vi "FlatToRichnixnet_grpc_DbMergeRequest.vi"(5 "OutputClusterType":T1, 11 "InputCluster":T3) -> (3 "OutputCluster":T1)   [LabVIEW 2025, in "xnet-grpc_client.lvlib"]
uses:
  nixnet_grpc_DbMergeRequest_Flat.ctl
  nidevice_grpc_Session_Flat.ctl
  nixnet_grpc_CopyMode.ctl
  nixnet_grpc_DbMergeRequest.ctl
  nixnet_grpc_DbMergeRequest_copy_mode_enum/nixnet_grpc_DbMergeRequest_copy_mode_enum.lvclass
  nidevice_grpc_Session.ctl
  xnet-grpc_client.lvlib
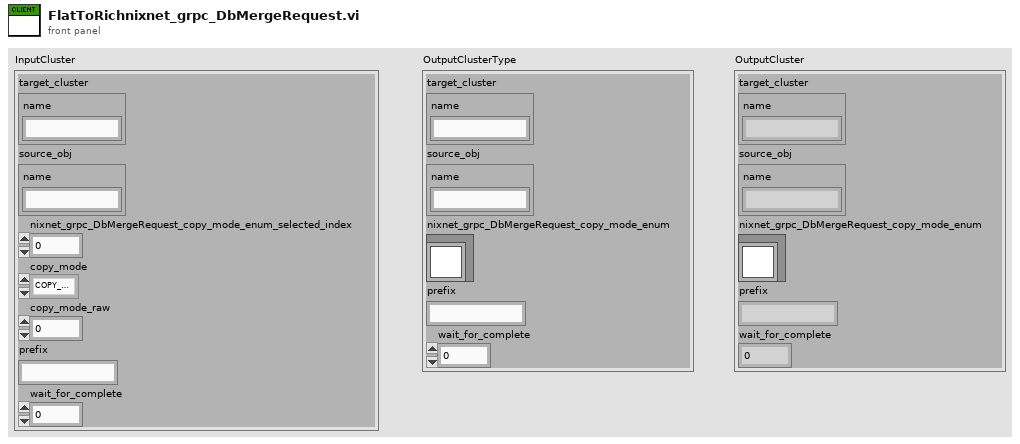
[diagram p1: front panel]
types:
  T1 = typedef "xnet-grpc_client.lvlib/nixnet_grpc_DbMergeRequest.ctl" = cluster{"target_cluster":T2, "source_obj":T2, "nixnet_grpc_DbMergeRequest_copy_mode_enum":refnum<class "nixnet_grpc_DbMergeRequest_copy_mode_enum.lvclass">, "prefix":string, "wait_for_complete":u32}
  T2 = typedef "xnet-grpc_client.lvlib/nidevice_grpc_Session.ctl" = cluster{"name":string}
  T3 = typedef "xnet-grpc_client.lvlib/nixnet_grpc_DbMergeRequest_Flat.ctl" = cluster{"target_cluster":T4, "source_obj":T4, "nixnet_grpc_DbMergeRequest_copy_mode_enum_selected_index":i32, "copy_mode":T5, "copy_mode_raw":u32, "prefix":string, "wait_for_complete":u32}
  T4 = typedef "xnet-grpc_client.lvlib/nidevice_grpc_Session_Flat.ctl" = cluster{"name":string}
  T5 = typedef "xnet-grpc_client.lvlib/nixnet_grpc_CopyMode.ctl" = enum32{"COPY_MODE_DB_MERGE_COPY_USE_SOURCE", "COPY_MODE_DB_MERGE_COPY_USE_TARGET", "COPY_MODE_DB_MERGE_MERGE_USE_SOURCE", "COPY_MODE_DB_MERGE_MERGE_USE_TARGET"}
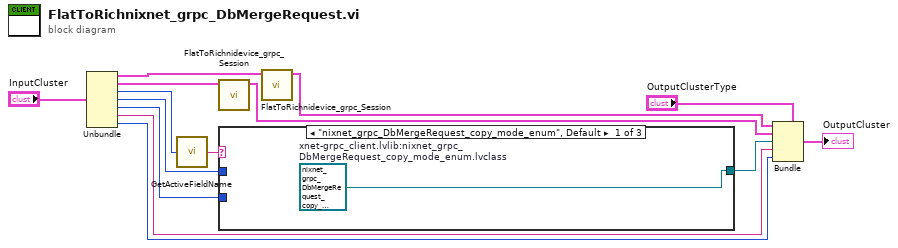
[diagram p0: block diagram]
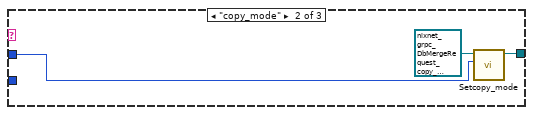
[diagram p2: hidden frame]
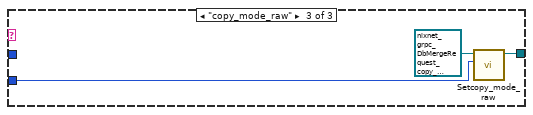
[diagram p3: hidden frame]
diagram:
  n1 = Unbundle "Unbundle"("InputCluster") -> ("target_cluster"=w11:T4, "source_obj"=w9:T4, "nixnet_grpc_DbMergeRequest_copy_mode_enum_selected_index"=w7:i32, "copy_mode"=w4:T5, "copy_mode_raw"=w3:u32, "prefix"=w2:string, "wait_for_complete"=w1:u32)
  n2 = call "GetActiveFieldName.vi"("protobuf index"=w7) -> ("oneof field name"=w6:string)
  n3 = call "FlatToRichnidevice_grpc_Session.vi"("InputCluster"=w9) -> ("OutputCluster"=w8:T2)  [unwired: 10 in]
  n4 = case "nixnet_grpc_DbMergeRequest_copy_mode_enum" shown="\"nixnet_grpc_DbMergeRequest_copy_mode_enum\", Default" w6 {
    tunnel: [w15 w17 w20] -> w5
    tunnel: w4 -> [_ w18 _]
    tunnel: w3 -> [_ _ w21]
    frame "nixnet_grpc_DbMergeRequest_copy_mode_enum", Default {
      w15 = refnum<class "nixnet_grpc_DbMergeRequest_copy_mode_enum.lvclass"> refnum  # xnet-grpc_client.lvlib:nixnet_grpc_DbMergeRequest_copy_mode_enum.lvclass
    }
    frame "copy_mode" {
      n5 = call "Setcopy_mode.vi"("Set_Val"=w18, "OneOfTemplate in"=refnum<class "nixnet_grpc_DbMergeRequest_copy_mode_enum.lvclass"> refnum) -> ("OneOfTemplate out"=w17:refnum<class "nixnet_grpc_DbMergeRequest_copy_mode_enum.lvclass">)  [unwired: 8 in, 1 out]
    }
    frame "copy_mode_raw" {
      n6 = call "Setcopy_mode_raw.vi"("Set_Val"=w21, "OneOfTemplate in"=refnum<class "nixnet_grpc_DbMergeRequest_copy_mode_enum.lvclass"> refnum) -> ("OneOfTemplate out"=w20:refnum<class "nixnet_grpc_DbMergeRequest_copy_mode_enum.lvclass">)  [unwired: 8 in, 1 out]
    }
  }
  n7 = call "FlatToRichnidevice_grpc_Session.vi"("InputCluster"=w11) -> ("OutputCluster"=w10:T2)  [unwired: 10 in]
  n8 = Bundle "Bundle"(cluster="OutputClusterType", "target_cluster"=w10, "source_obj"=w8, "nixnet_grpc_DbMergeRequest_copy_mode_enum"=w5, "prefix"=w2, "wait_for_complete"=w1) -> (→"OutputCluster":T1)
